vi "CMD_SERIALOPEN.vi"(6 "Gantry in":refnum<class "Gantry.lvclass">, 7 "Console Log in":refnum<class "Console Log.lvclass">, 8 "error in (no error)":errorcluster, 10 "Arguments":string[](array[string]), 11 "gScript Interpreter in":refnum<class "gScript Interpreter.lvclass">) -> (0 "error out":errorcluster, 3 "gScript Interpreter out":refnum<class "gScript Interpreter.lvclass">, 4 "Gantry out":refnum<class "Gantry.lvclass">, 5 "Console Log out":refnum<class "Console Log.lvclass">)   [LabVIEW 2024, in "gScript Interpreter.lvclass"]
uses:
  gScript Interpreter.lvclass
  Shared Components/Gantry Class/Gantry.lvclass
  Application Utilities/Console Log/Console Log.lvclass
  Shared Components/FlexWorktable/FlexWorktable.lvclass
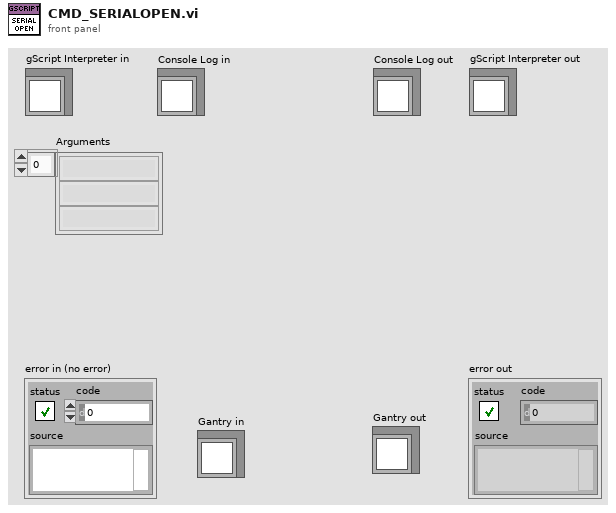
[diagram p1: front panel]
types:
  T1 = typedef "Serial Configuration.ctl" = cluster{"timeout ms":u32, "data bits":u16, "parity":enum16{"None", "Odd", "Even", "Mark", "Space"}, "baud rate":u32, "stop bits":u16, "flow control":u16}
  T2 = typedef "Memory Cell.ctl" = cluster{"type":T3, "x":dbl, "y":dbl, "z":dbl, "w":dbl}
  T3 = typedef "Memory Cell Type Enum.ctl" = enum16{"integer", "float", "vector", "rotation"}
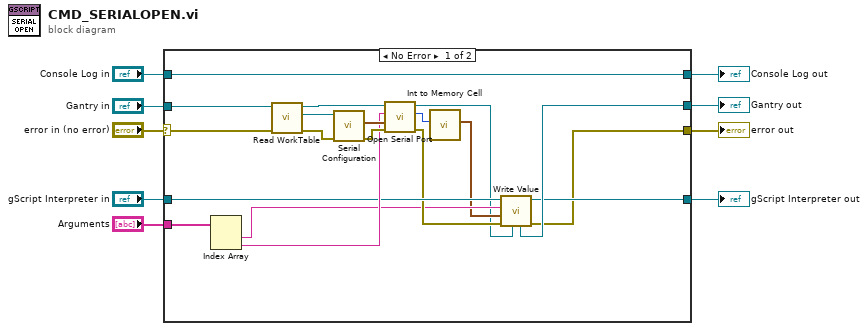
[diagram p0: block diagram]
diagram:
  n1 = case shown="No Error" "error in (no error)" {
    selector: "error in (no error)" -> [w26 w32]
    tunnel: [w10 w32] -> w8
    tunnel: [w11 w31] -> w6
    tunnel: "gScript Interpreter in" -> [w18 w31]
    tunnel: "Arguments" -> [w20 _]
    tunnel: "Gantry in" -> [w27 w30]
    tunnel: [w12 w30] -> w3
    tunnel: "Console Log in" -> [w28 w29]
    tunnel: [w28 w29] -> w1
    frame No Error {
      n2 = Index Array(array=w20) -> (element #1=w16:string, element #2=w19:string)  [unwired: 2 in]
      n3 = call-dynamic "Read WorkTable.vi"("error in"=w26, "Gantry Class in"=w27) -> ("error out"=w24:errorcluster, "Worktable"=w25:refnum<class "FlexWorktable.lvclass">, "Gantry Class out"=w23:refnum<class "Gantry.lvclass">)  [unwired: 7 in]
      n4 = call "Serial Configuration.vi"("error in (no error)"=w24, "FlexWorktable in"=w25) -> ("error out"=w22:errorcluster, "Serial Configuration"=w21:T1)  [unwired: 7 in, 1 out]
      n5 = call "Open Serial Port.vi"("error in (no error)"=w22, "Serial Configuraiton"=w21, "VISA resource"=w19, "Gantry in"=w23) -> ("error out"=w17:errorcluster, "Connection ID"=w15:i32, "Gantry out"=w13:refnum<class "Gantry.lvclass">)  [unwired: 5 in]
      n6 = call "Int to Memory Cell.vi"("Numeric"=w15) -> ("Memory Cell"=w14:T2)  [unwired: 10 in]
      n7 = call-dynamic "Write Value.vi"("Gantry in"=w13, "error in (no error)"=w17, "Value"=w14, "Address"=w16, "gScript Interpreter in"=w18) -> ("error out"=w10:errorcluster, "gScript Interpreter out"=w11:refnum<class "gScript Interpreter.lvclass">, "Gantry out"=w12:refnum<class "Gantry.lvclass">)  [unwired: 4 in]
    }
    frame Error {
    }
  }
  "error out" <- w8
  "gScript Interpreter out" <- w6
  "Gantry out" <- w3
  "Console Log out" <- w1
